vi "getOptions.vi"(8 "error in (no error)":errorcluster, 11 "tBSONRegEx in":refnum<class "tBSONRegEx.lvclass">) -> (0 "error out":errorcluster, 2 "Options":T1, 3 "tBSONRegEx out":refnum<class "tBSONRegEx.lvclass">)   [LabVIEW 2013, in "BSON.lvlib" / "tBSONRegEx.lvclass"]
uses:
  tBSONRegEx.lvclass
  options.ctl
  tBSONRegEx.lvclass/tBSONRegEx.ctl
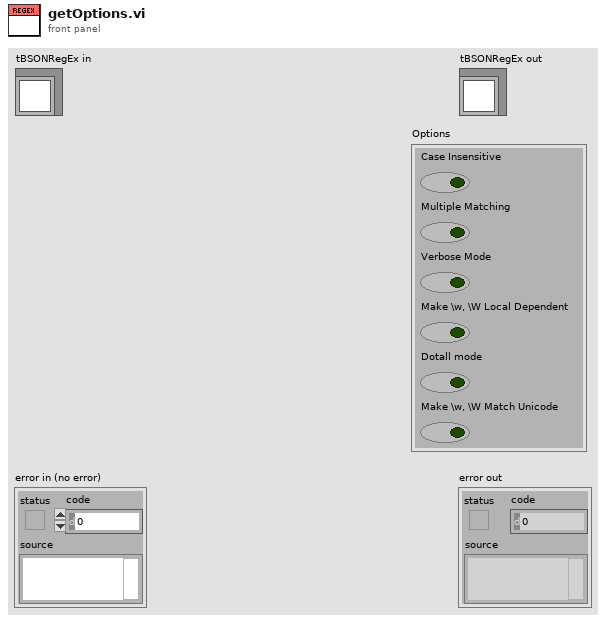
[diagram p1: front panel]
types:
  T1 = typedef "BSON.lvlib/tBSONRegEx.lvclass/options.ctl" = cluster{"Case Insensitive":bool, "Multiple Matching":bool, "Verbose Mode":bool, "Make \\w, \\W Local Dependent":bool, "Dotall mode":bool, "Make \\w, \\W Match Unicode":bool}
  T2 = cluster{"Case Insensitive":bool, "Multiple Matching":bool, "Verbose Mode":bool, "Make \\w, \\W Local Dependent":bool, "Dotall mode":bool, "Make \\w, \\W Match Unicode":bool}
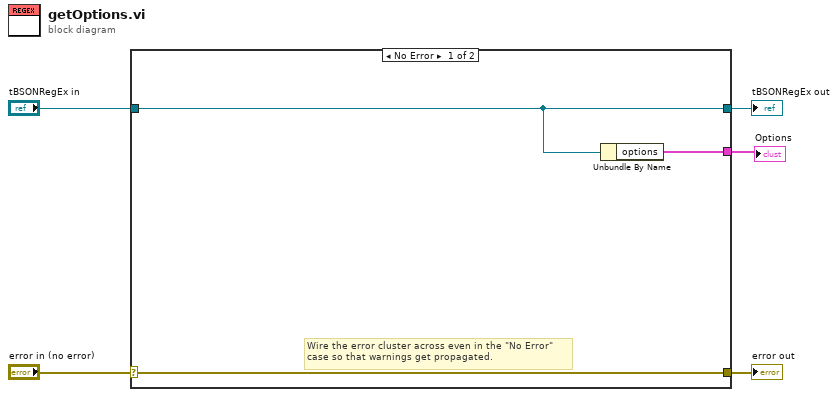
[diagram p0: block diagram]
diagram:
  n1 = case shown="No Error" "error in (no error)" {
    selector: "error in (no error)" -> [w8 w10]
    tunnel: [w8 w10] -> w4
    tunnel: [w7 w9] -> w2
    tunnel: "tBSONRegEx in" -> [w7 w9]
    tunnel: [w6 _] -> w1
    frame No Error {
      # "Wire the error cluster across even in the \"No Error\"\ncase so that warnings get propagated."
      n2 = Unbundle By Name(w7) -> ("options"=w6:T2)
    }
    frame Error {
    }
  }
  "error out" <- w4
  "tBSONRegEx out" <- w2
  "Options" <- w1
